vi "Fetch Measurement (Occupied Bandwidth).vi"(0 "VISA resource name":refnum<visa-resource-name>, 5 "Timeout (10000 ms)":i32=10000 format="%.0g", 11 "error in (no error)":errorcluster) -> (2 "Transmit Frequency Error Hz":dbl, 3 "Res BW":dbl, 4 "VISA resource name out":refnum<visa-resource-name>, 6 "Occupied Bandwidth":dbl, 8 "Spectrum Trace Points":dbl, 10 "Total Power":dbl, 13 "X DB Bandwidth":dbl, 14 "Span":dbl, 15 "error out":errorcluster)   [LabVIEW 2018, in "Agilent MXA Series.lvlib"]
doc: "Returns the results of last measurement(Occupied Bandwidth) and does not initiate data acquisition.\n\n<B>Note:</B>\n\nUse this VI only with other low-level VIs. The high-level VIs automatically incorporate this functionality. This VI does not check the instrument status."
uses:
  Agilent MXA Series.lvlib
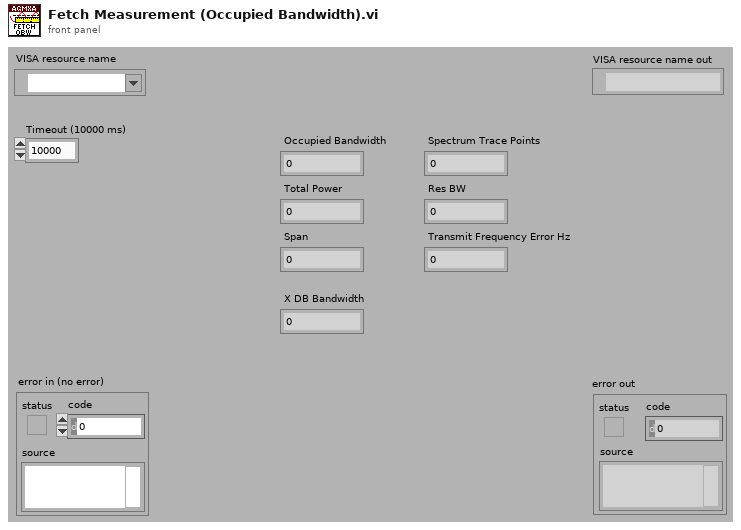
[diagram p1: front panel]
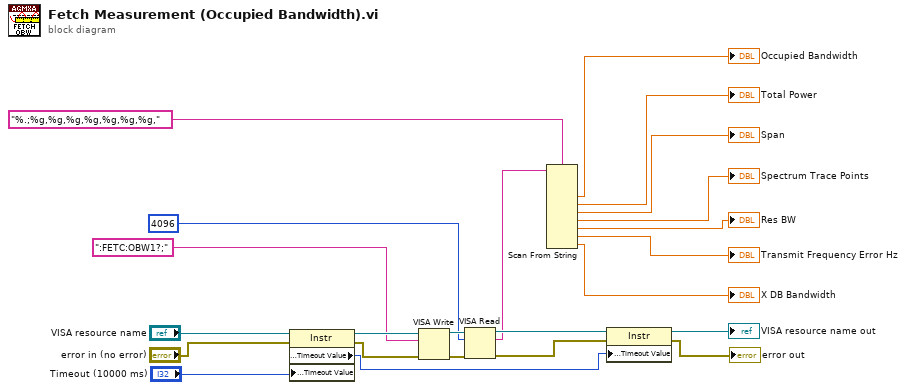
[diagram p0: block diagram]
diagram:
  n1 = property on="Property Node" class="Instr"(reference="VISA resource name", error in="error in (no error)", "General Settings:Timeout Value"="Timeout (10000 ms)") -> (reference out=w17:refnum<visa-resource-name>, error out=w18:errorcluster, "General Settings:Timeout Value"=w1:u32)
  n2 = VISA Write(VISA resource name=w17, write buffer=":FETC:OBW1?;", error in (no error)=w18) -> (VISA resource name out=w15:refnum<visa-resource-name>, error out=w16:errorcluster)  [unwired: 1 out]
  n3 = VISA Read(VISA resource name=w15, byte count=4096, error in (no error)=w16) -> (VISA resource name out=w11:refnum<visa-resource-name>, read buffer=w10:string, error out=w12:errorcluster)  [unwired: 1 out]
  n4 = Scan From String(format string="%.;%g,%g,%g,%g,%g,%g,%g,", input string=w10) -> (output 1=→"Occupied Bandwidth":dbl, output 2=→"Total Power":dbl, output 3=→"Span":dbl, output 4=→"Spectrum Trace Points":dbl, output 5=→"Res BW":dbl, output 6=→"Transmit Frequency Error Hz":dbl, output 7=→"X DB Bandwidth":dbl)  [unwired: 9 in, 3 out]
  n5 = property on="Property Node" class="Instr"(reference=w11, error in=w12, "General Settings:Timeout Value"=w1) -> (reference out=→"VISA resource name out":refnum<visa-resource-name>, error out=→"error out":errorcluster)
